vi "Config Display.vi"(0 "VISA resource name":refnum<visa-resource-name>, 1 "Element (1: Element 1)":u16(ring)=1 items=["", "Element1", "Element2", "Element3", "Sigma"], 5 "Display (1: A)":u16(ring)=1 items=["", "A", "B", "C"], 7 "Harmonics Mode (F: Normal)":bool, 9 "Resolution (0: Low)":u16(ring) items=["Low", "High"], 11 "error in (no error)":errorcluster, 12 "Normal Function (0: V)":u16(ring) items=["V", "A", "W", "VA", "var", "PF", "deg", "Vpk", "Apk", "V Hz", "A Hz", "Wh", "Wh+", "Wh-", "Ah", "Ah+", "Ah-", "Math", "Time"], 13 "Harmonics Function (0: V)":u16(ring) items=["V", "A", "W", "PF", "V Hz", "A Hz", "VTHD", "ATHD", "Vcon", "Acon", "Wcon", "Vdeg", "Adeg", "Order"], 14 "Display Order (1)":u8=1 min=1 max=50) -> (4 "VISA resource name out":refnum<visa-resource-name>, 15 "error out":errorcluster)   [LabVIEW 2016, in "Yokogawa WT200 Series.lvlib"]
doc: "This VI sends the Display Configuration commands to the WT200 Series."
uses:
  Yokogawa WT200 Series.lvlib
panel:
  # "Harmonics\nNormal"
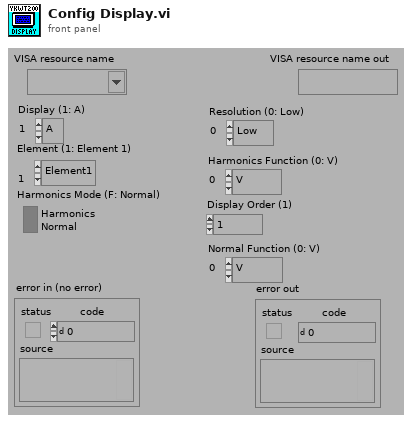
[diagram p1: front panel]
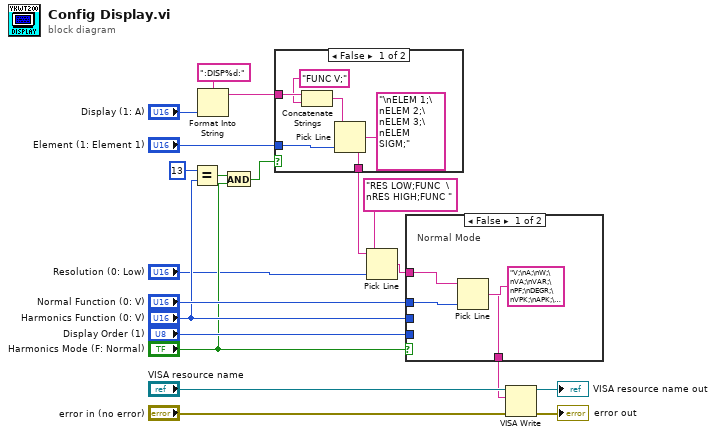
[diagram p0: block diagram]
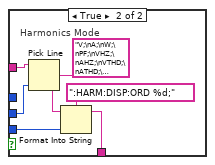
[diagram p3: hidden frame]
diagram:
  n1 = Equal?(x=u16 13, y="Harmonics Function (0: V)") -> (x = y?=w9:bool)
  n2 = Format Into String(format string=":DISP%d:", "Display (1: A)") -> (resulting string=w6:string)  [unwired: 2 in, 1 out]
  n3 = And(x=w9, y="Harmonics Mode (F: Normal)") -> (x .and. y?=w7:bool)
  n4 = case shown="False" w7 {
    tunnel: "Element (1: Element 1)" -> [w25 _]
    tunnel: w6 -> [w23 w27]
    tunnel: [w24 w27] -> w3
    frame False {
      n5 = Concatenate Strings(w23, "FUNC V;") -> (w22:string)
      n6 = Pick Line(string ("")=w22, multi-line string="\nELEM 1;\nELEM 2;\nELEM 3;\nELEM SIGM;" ("ÏÙÁ×²Ý•¶Žš—ñ"), line index=w25) -> (output string=w24:string)
    }
    frame True {
      # "Harmonics, Order"
    }
  }
  n7 = Pick Line(string ("")=w3, multi-line string="RES LOW;FUNC  \nRES HIGH;FUNC ", line index="Resolution (0: Low)") -> (output string=w2:string)
  n8 = case shown="False" "Harmonics Mode (F: Normal)" {
    tunnel: "Normal Function (0: V)" -> [w30 _]
    tunnel: [w29 w35] -> w5
    tunnel: "Harmonics Function (0: V)" -> [_ w37]
    tunnel: "Display Order (1)" -> [_ w36]
    tunnel: w2 -> [w28 w32]
    frame False {
      # "Normal Mode"
      n9 = Pick Line(string ("")=w28, multi-line string="V;\nA;\nW;\nVA;\nVAR;\nPF;\nDEGR;\nVPK;\nAPK;\nVHZ;\nAHZ;\nWH;\nWHP;\nWHM;\nAH;\nAHP;\nAHM;\nMATH;\nTIME;", line index=w30) -> (output string=w29:string)
    }
    frame True {
      # "Harmonics Mode"
      n10 = Pick Line(string ("")=w32, multi-line string="V;\nA;\nW;\nPF;\nVHZ;\nAHZ;\nVTHD;\nATHD;\nVCON;\nACON;\nWCON;\nVDEG;\nADEG;\nORD;", line index=w37) -> (output string=w34:string)
      n11 = Format Into String(format string=":HARM:DISP:ORD %d;", initial string=w34, w36) -> (resulting string=w35:string)  [unwired: 1 in, 1 out]
    }
  }
  n12 = VISA Write(VISA resource name="VISA resource name", write buffer=w5, error in (no error)="error in (no error)") -> (VISA resource name out=→"VISA resource name out":refnum<visa-resource-name>, error out=→"error out":errorcluster)  [unwired: 1 out]
